vi "SingleShot.vi"(8 "error in (no error)":errorcluster, 11 "CameraTesting in":refnum<class "CameraTesting.lvclass">) -> (0 "error out":errorcluster, 3 "CameraTesting out":refnum<class "CameraTesting.lvclass">)   [LabVIEW 2020, in "CameraTesting.lvlib" / "CameraTesting.lvclass"]
uses:
  CameraTesting.lvclass
  CameraTesting.lvclass/CameraTesting.ctl
  Camera/ICamera/ICamera/ICamera.lvclass
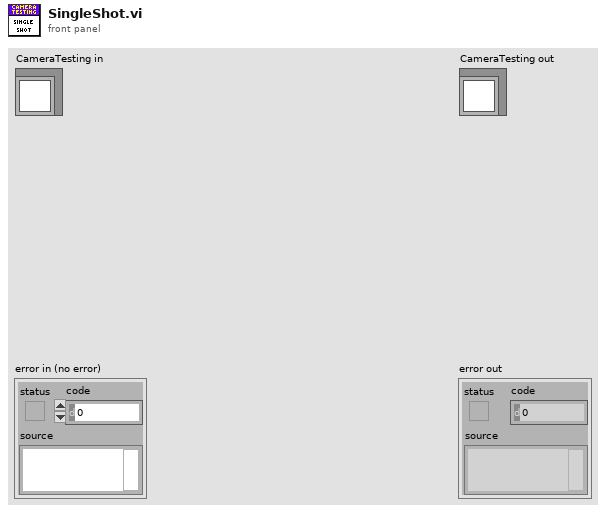
[diagram p1: front panel]
types:
  T1 = typedef "ICameraTesting.lvlib/ICameraTesting.lvclass/StatusUpdated.ctl" = refnum<user-event>
  T2 = typedef "ICamera.lvlib/ICamera.lvclass/SnapInfo.ctl" = cluster{"image depth":i32, "PixelData":u8[], "Bounds":cluster{"Height":i16, "Width":i16}}
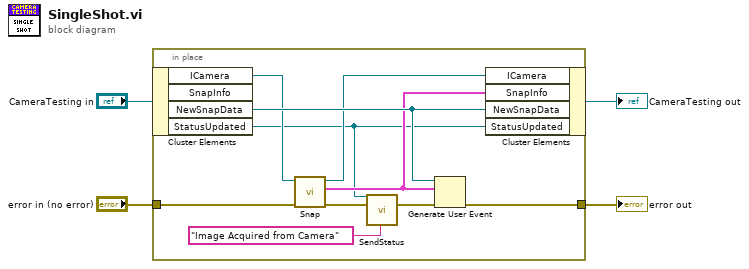
[diagram p0: block diagram]
diagram:
  n1 = in-place {
    in-place-border: "error in (no error)" -> [w14]
    in-place-border: [w13] -> w1
    n2 = in-place-cluster #1("CameraTesting in") -> ("ICamera"=w10:refnum<class "ICamera.lvclass">, "NewSnapData"=w12:refnum<user-event>, "StatusUpdated"=w5:T1)  [unwired: 1 out]
    n3 = call-dynamic "Snap.vi"("error in (no error)"=w14, "ICamera in"=w10) -> ("error out"=w7:errorcluster, "SnapInfo"=w11:T2, "ICamera out"=w9:refnum<class "ICamera.lvclass">)  [unwired: 7 in]
    n4 = call "SendStatus.vi"("StatusUsrEvn"=w5, "error in"=w7, "Text"="Image Acquired from Camera") -> ("error out"=w6:errorcluster)  [unwired: 24 in]
    n5 = Generate User Event(user event=w12, event data cluster=w11, error in=w6) -> (error out=w13:errorcluster)  [unwired: 1 in, 1 out]
    n6 = in-place-cluster #1("ICamera"=w9, "SnapInfo"=w11, "NewSnapData"=w12, "StatusUpdated"=w5) -> (→"CameraTesting out":refnum<class "CameraTesting.lvclass">)
  }
  "error out" <- w1
